vi "HRM-Stage4-init_main.vi"() -> (0 "error out":errorcluster, 3 "Init cluster":T1)   [LabVIEW 2020]
uses:
  Stage 3/HRM-Stage3-User_events.ctl
  Stage 3/HRM-Stage3-init_cluster.ctl
  HRM-Stage4-User_events.ctl
  HRM-Stage4-init_cluster.ctl
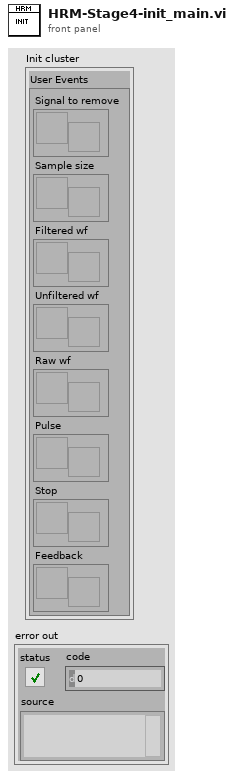
[diagram p1: front panel]
types:
  T1 = typedef "HRM-Stage4-init_cluster.ctl" = cluster{"User Events":T2}
  T2 = typedef "HRM-Stage4-User_events.ctl" = cluster{"Signal to remove":refnum<user-event>, "Sample size":refnum<user-event>, "Filtered wf":refnum<user-event>, "Unfiltered wf":refnum<user-event>, "Raw wf":refnum<user-event>, "Pulse":refnum<user-event>, "Stop":refnum<user-event>, "Feedback":refnum<user-event>}
  T3 = typedef "HRM-Stage3-init_cluster.ctl" = cluster{"User events":T4}
  T4 = typedef "HRM-Stage3-User_events.ctl" = cluster{"Signal to remove":refnum<user-event>, "Sample size":refnum<user-event>, "Filtered wf":refnum<user-event>, "Unfiltered wf":refnum<user-event>, "Raw wf":refnum<user-event>, "Pulse":refnum<user-event>, "Stop":refnum<user-event>}
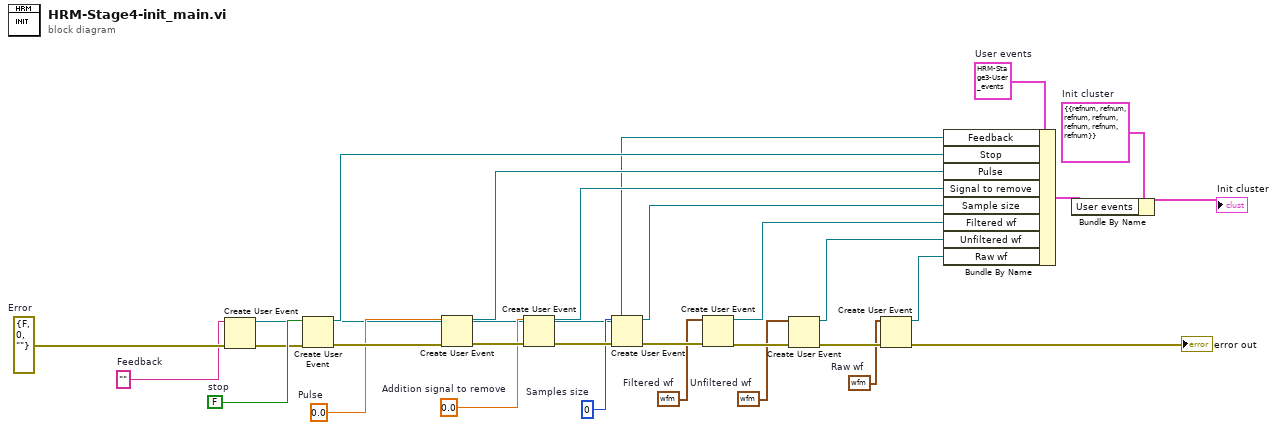
[diagram p0: block diagram]
diagram:
  w3 = ""  # Feedback
  w4 = errorcluster {"status"=FALSE, "code"=0, "source"=""}  # Error
  w26 = FALSE  # stop
  w24 = T3 {"User events"={"Signal to remove"=refnum, "Sample size"=refnum, "Filtered wf"=refnum, "Unfiltered wf"=refnum, "Raw wf"=refnum, "Pulse"=refnum, "Stop"=refnum}}  # Init cluster
  w21 = 0.0  # Pulse
  w15 = T4 {"Signal to remove"=refnum, "Sample size"=refnum, "Filtered wf"=refnum, "Unfiltered wf"=refnum, "Raw wf"=refnum, "Pulse"=refnum, "Stop"=refnum}  # User events
  w10 = 0  # Samples size
  w9 = 0.0  # Addition signal to remove
  w8 = waveform(dbl) {"t0"=timestamp(0 s since 1904-01-01), "dt"=1.0, "Y"=[]}  # Filtered wf
  w7 = waveform(dbl) {"t0"=timestamp(0 s since 1904-01-01), "dt"=1.0, "Y"=[]}  # Unfiltered wf
  w6 = waveform(dbl) {"t0"=timestamp(0 s since 1904-01-01), "dt"=1.0, "Y"=[]}  # Raw wf
  n1 = Create User Event(user event datatype=w3, error in=w4) -> (user event=w2:refnum<user-event>, error out=w5:errorcluster)
  n2 = Create User Event(user event datatype=w26, error in=w5) -> (user event=w28:refnum<user-event>, error out=w27:errorcluster)
  n3 = Create User Event(user event datatype=w21, error in=w27) -> (user event=w22:refnum<user-event>, error out=w23:errorcluster)
  n4 = Create User Event(user event datatype=w9, error in=w23) -> (user event=w16:refnum<user-event>, error out=w14:errorcluster)
  n5 = Create User Event(user event datatype=w10, error in=w14) -> (user event=w17:refnum<user-event>, error out=w13:errorcluster)
  n6 = Create User Event(user event datatype=w8, error in=w13) -> (user event=w18:refnum<user-event>, error out=w12:errorcluster)
  n7 = Create User Event(user event datatype=w7, error in=w12) -> (user event=w19:refnum<user-event>, error out=w11:errorcluster)
  n8 = Create User Event(user event datatype=w6, error in=w11) -> (user event=w20:refnum<user-event>, error out=→"error out":errorcluster)
  n9 = Bundle By Name(cluster=w15, "Feedback"=w2, "Stop"=w28, "Pulse"=w22, "Signal to remove"=w16, "Sample size"=w17, "Filtered wf"=w18, "Unfiltered wf"=w19, "Raw wf"=w20) -> (w25:T4)
  n10 = Bundle By Name(cluster=w24, "User events"=w25) -> (→"Init cluster":T3)
